vi "Process Incoming Frames.vi"(7 "Incoming Session":refnum<k21>, 8 "error in":errorcluster, 9 "Incoming Signal Info":T4 {"Signal Settings Out"."Protection Configuration"."CRC Channels"."Data Type" items=["Signed", "Unsigned", "IEEE Float"]}, 10 "Incoming RT Data Refs":T2, 11 "Incoming Frame Info In":T1) -> (0 "error out":errorcluster, 1 "Incoming Signal Info Out":T4 {"Signal Settings Out"."Protection Configuration"."CRC Channels"."Data Type" items=["Signed", "Unsigned", "IEEE Float"]}, 3 "Incoming Frame Info Out":T1, 5 "session out":refnum<k21>)   [LabVIEW 2019]
doc: "This example demonstrates receiving automatically converted values of signals, along with the associated timestamp value, using an NI-XNET Signal Input XY session. \n\nThis example can run against the CAN Signal Output XY example, assuming you have a properly terminated CAN cable connected to two CAN ports.\n\nIf you have no database aliases on your system, the example automatically loads the nixnet_example database."
uses:
  Types/Incoming Frame Info.ctl
  SubModules/Frame-Protection-Support/Source/Shared/Types/RT_Incoming_Signal_Info.ctl
  SubModules/Frame-Protection-Support/Source/Shared/Types/RT Exported Signal Settings.ctl
  SubModules/Frame-Protection-Support/Source/Shared/Types/Exported Counter Settings.ctl
  SubModules/Frame-Protection-Support/Source/Engine/Types/RT Protection Configuration.ctl
  SubModules/Frame-Protection-Support/Source/Shared/Types/Protection Type.ctl
  SubModules/Frame-Protection-Support/Source/Shared/Types/XNET Signal Configuration.ctl
  Types/Incoming Signal RT Data References.ctl
  <vilib>/NI/NIVS Inline Async API/_Data Access Engine/Data Access Engine/Types/Write.DVR.ctl
  <vilib>/NI/NIVS Inline Async API/_Data Access Engine/Access Type Classes/Write/Write.lvclass
  <vilib>/NI/NIVS Inline Async API/_Data Access Engine/Access Type Classes/Write/Write.lvclass/Write.ctl
  <vilib>/NI/NIVS Inline Async API/_Data Access Engine/Data Access Engine/Methods/Write.Data.vi
  SubModules/Frame-Protection-Support/Source/Engine/SubVIs/Get Protection Signals.vi
  <vilib>/NI/NIVS Inline Async API/_Data Access Engine/Access Type Classes/Write/Write.ProcessData.vi
  <vilib>/NI/NIVS Inline Async API/_Data Access Engine/Access Type Classes/Write/Write.Buffer.vi
  <vilib>/NI/NIVS Inline Async API/_Data Access Engine/Access Type Classes/Write/Write.Commit.vi
  <vilib>/xnet/xnet.llb/XNET Read (Signal XY).vi
  <vilib>/xnet/xnet.llb/XNET Convert.vi
  <vilib>/xnet/xnet.llb/XNET Convert (Signal to Frame Raw).vi
  <vilib>/NI/NIVS Inline Async API/_Data Access Engine/Data Access Engine/Data Access Engine.lvclass
  <vilib>/NI VeriStand/Custom Device Tools/Custom Device Utility Library/Custom Device Utility Library.lvlib
  SubModules/Frame-Protection-Support/Source/Engine/Protection and Counter Support Engine.lvlib
  SubModules/Frame-Protection-Support/Source/Shared/Protection and Counter Support Shared.lvlib
panel:
  out "data 2":T10(array[cluster])
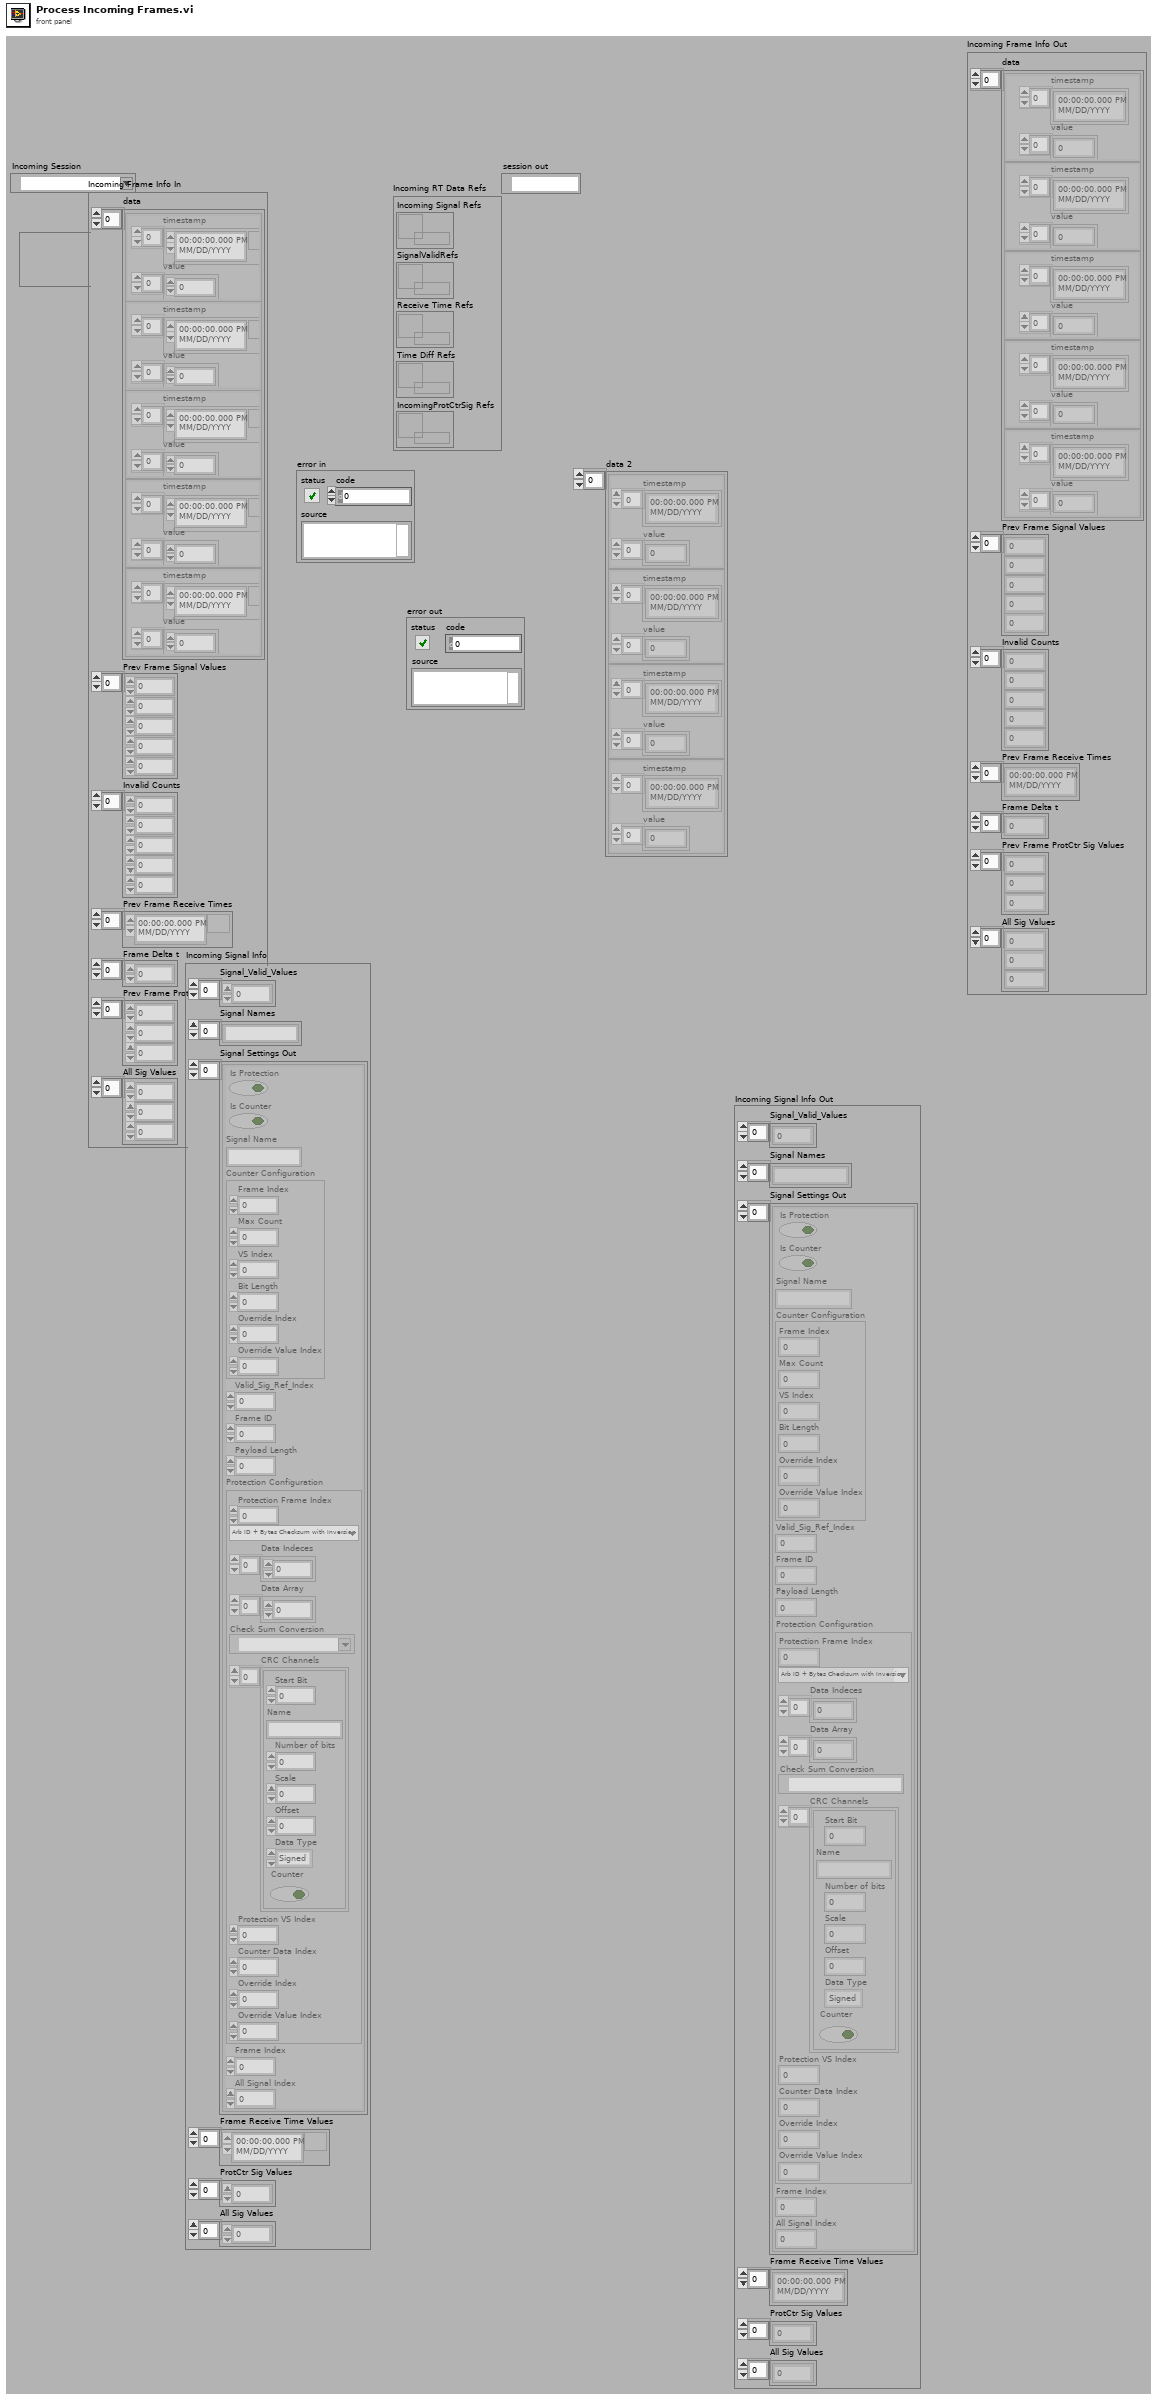
[diagram p1: front panel]
types:
  T1 = typedef "Incoming Frame Info.ctl" = cluster{"data":cluster{"timestamp":timestamp[], "value":dbl[]}[], "Prev Frame Signal Values":dbl[], "Invalid Counts":dbl[], "Prev Frame Receive Times":timestamp[], "Frame Delta t":dbl[], "Prev Frame ProtCtr Sig Values":dbl[], "All Sig Values":dbl[]}
  T2 = typedef "Incoming Signal RT Data References.ctl" = cluster{"Incoming Signal Refs":T3, "SignalValidRefs":T3, "Receive Time Refs":T3, "Time Diff Refs":T3, "IncomingProtCtrSig Refs":T3}
  T3 = typedef "Data Access Engine.lvlib/Data Access Engine.lvclass/Write.DVR.ctl" = refnum<data-value>
  T4 = typedef "RT_Incoming_Signal_Info.ctl" = cluster{"Signal_Valid_Values":dbl[], "Signal Names":string[], "Signal Settings Out":T5[], "Frame Receive Time Values":timestamp[], "ProtCtr Sig Values":dbl[], "All Sig Values":dbl[]}
  T5 = typedef "RT Exported Signal Settings.ctl" = cluster{"Is Protection":bool, "Is Counter":bool, "Signal Name":string, "Counter Configuration":T6, "Valid_Sig_Ref_Index":i32, "Frame ID":u32, "Payload Length":u32, "Protection Configuration":T7, "Frame Index":i32, "All Signal Index":i32}
  T6 = typedef "Protection and Counter Support Shared.lvlib/Exported Counter Settings.ctl" = cluster{"Frame Index":i32, "Max Count":dbl, "VS Index":i32, "Bit Length":i64, "Override Index":i32, "Override Value Index":i32}
  T7 = typedef "Protection and Counter Support Engine.lvlib/RT Protection Configuration.ctl" = cluster{"Protection Frame Index":i32, "Protection Type":T8, "Data Indeces":i32[], "Data Array":dbl[], "Check Sum Conversion":refnum<k21>, "CRC Channels":T9[], "Protection VS Index":i32, "Counter Data Index":i32, "Override Index":i32, "Override Value Index":i32}
  T8 = typedef "Protection and Counter Support Shared.lvlib/Protection Type.ctl" = enum16{"Arb ID + Bytes Checksum with Inversion", "Arb ID + Bytes CRC with Inversion", "Reversed Raw Signal Checksum with Inversion", "Concatenated Two's Compliment"}
  T9 = typedef "Protection and Counter Support Shared.lvlib/XNET Signal Configuration.ctl" = cluster{"Start Bit":i32, "Name":string, "Number of bits":i32, "Scale":dbl, "Offset":dbl, "Data Type":u32, "Counter":bool}
  T10 = cluster{"timestamp":timestamp[], "value":dbl[]}[]
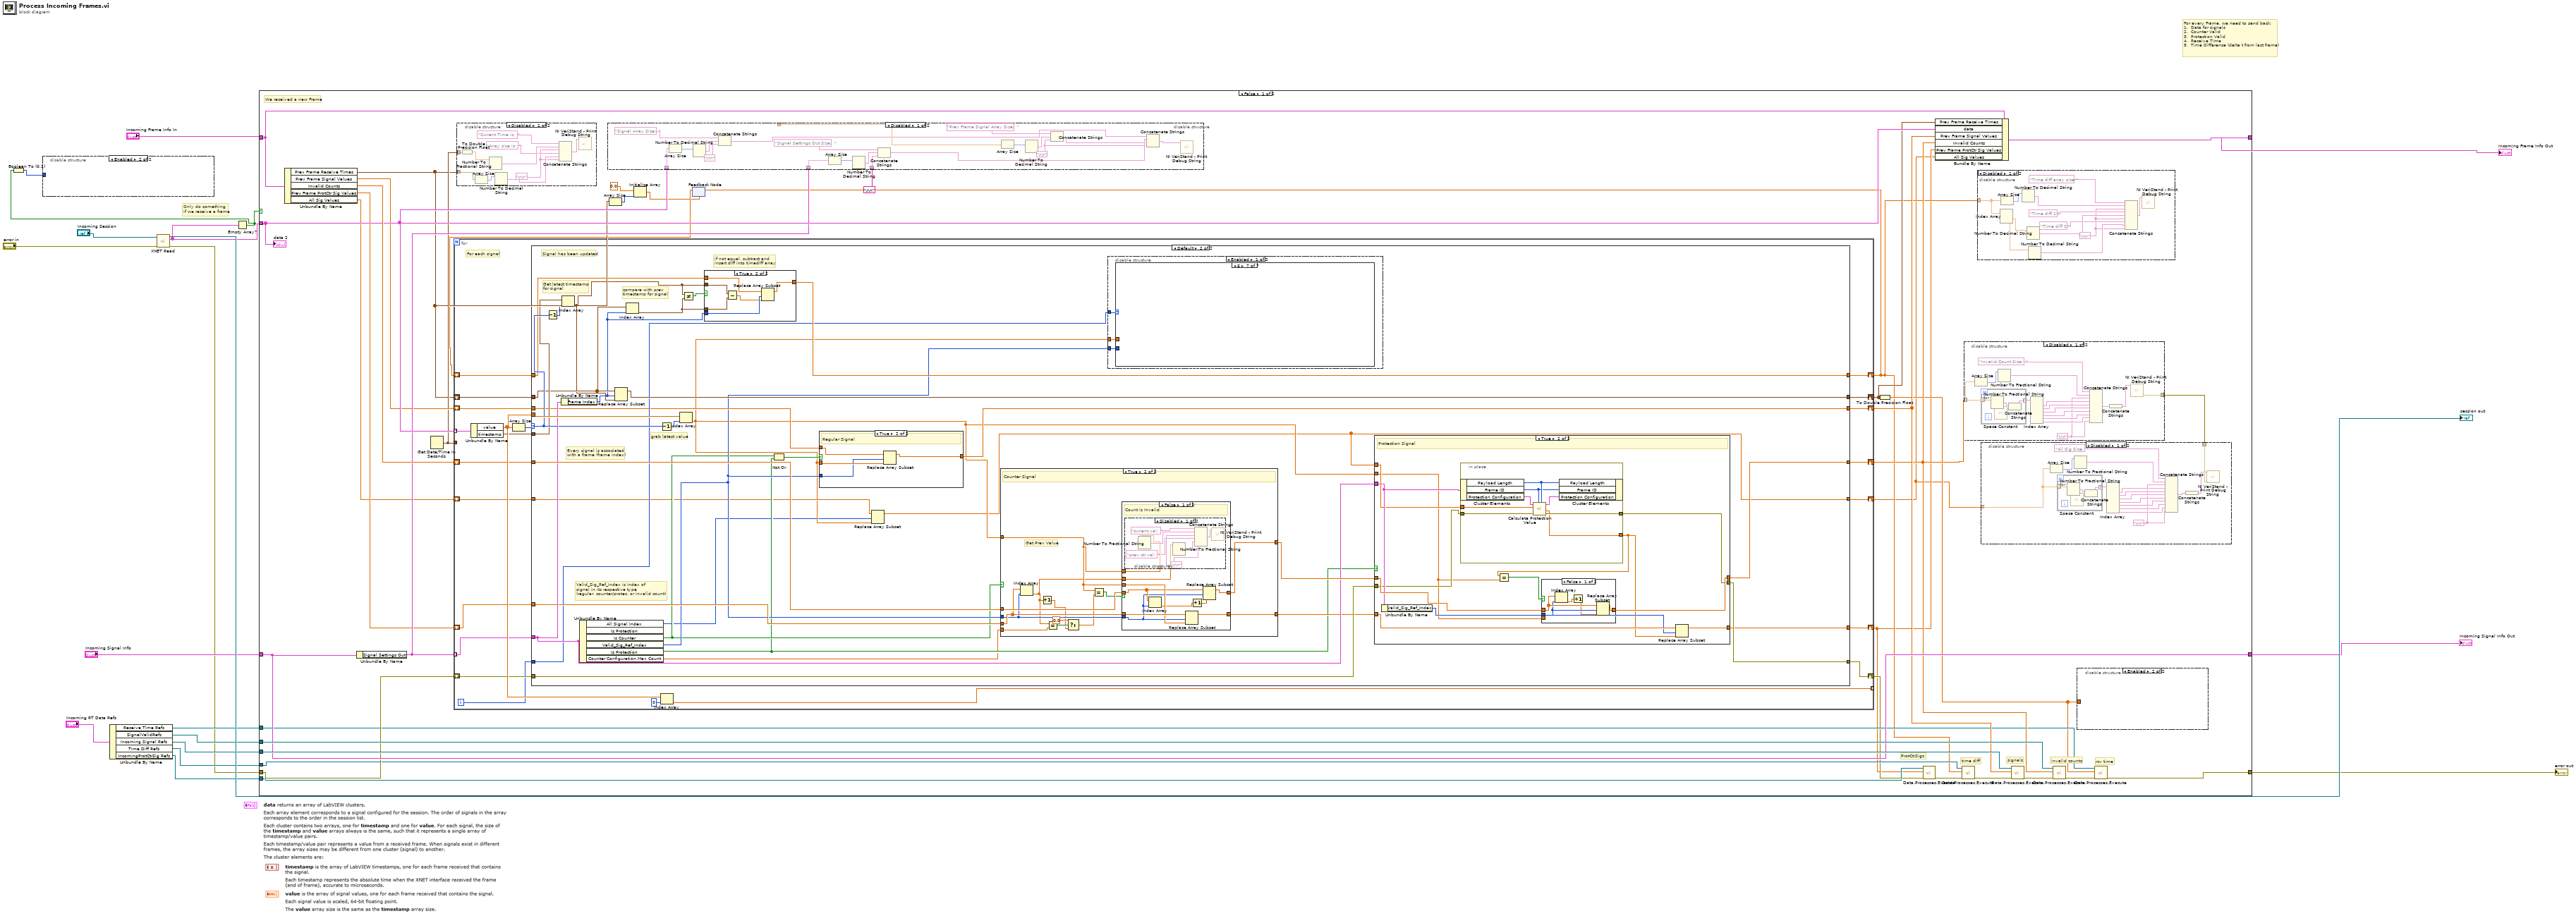
[diagram p0: block diagram]
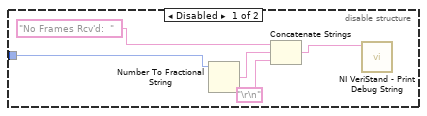
[diagram p2: hidden frame]
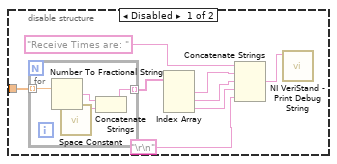
[diagram p7: hidden frame]
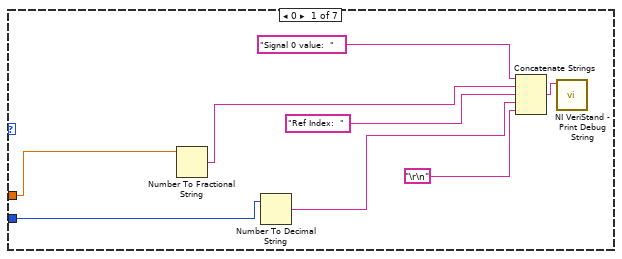
[diagram p11: hidden frame]
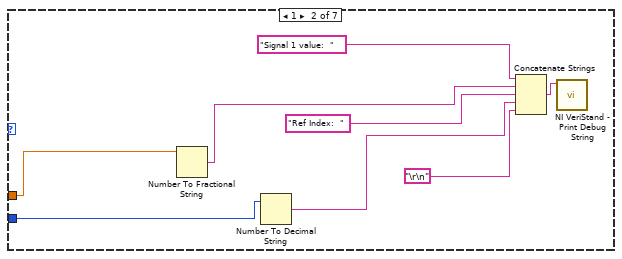
[diagram p12: hidden frame]
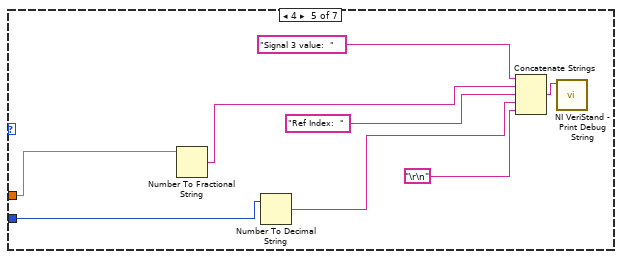
[diagram p15: hidden frame]
diagram:
  # "Only do something\nif we receive a frame"
  # "For every Frame, we need to send back:\n1.  Data for signals\n2.  Counter Valid\n3.  Protection Valid\n4.  Receive Time\n5.  Time Difference (delta t from last frame)"
  n1 = Unbundle By Name("Incoming RT Data Refs") -> ("Receive Time Refs"=w10:T3, "SignalValidRefs"=w9:T3, "Incoming Signal Refs"=w8:T3, "Time Diff Refs"=w4:T3, "IncomingProtCtrSig Refs"=w3:T3)
  n2 = call-poly <vilib>:"XNET Read.vi"("session in"="Incoming Session", "error in (no error)"="error in") -> ("session out"=→"session out":refnum<k21>, "data"=w12:T10, "error out"=w1:errorcluster)  [unwired: 11 out]
  n3 = Empty Array?(array=w12) -> (empty?=w5:bool)
  n4 = Boolean To (0,1)(Boolean=w5) -> (0, 1=w6:i16)
  n5 = disable-structure shown="Enabled" {
    disable-tunnel: w6 -> [w19 _]
    frame Disabled {
      n6 = Number To Fractional String(number=w19) -> (F-format string=w22:string)  [unwired: 3 in]
      n7 = Concatenate Strings("No Frames Rcv'd:  ", w22, "\r\n") -> (w20:string)
      n8 = call <vilib>:"NI VeriStand - Print Debug String.vi"("Message"=w20) -> ()  [unwired: 10 in, 1 out]
    }
    frame Enabled {
    }
  }
  n9 = case shown="False" w5 {
    tunnel: w12 -> [w49 _]
    tunnel: w1 -> [w52 w323]
    tunnel: [w44 w323] -> w15
    tunnel: "Incoming Frame Info In" -> [w55 w322]
    tunnel: [w59 w322] -> w7
    tunnel: w8 -> [w57 _]
    tunnel: w9 -> [w56 _]
    tunnel: "Incoming Signal Info" -> [w54 w321]
    tunnel: [w54 w321] -> w13
    tunnel: w10 -> [w43 _]
    tunnel: w4 -> [w38 _]
    tunnel: w3 -> [w29 _]
    frame False {
      # "ProtCtrSigs"
      # "time diff"
      # "signals"
      # "invalid counts"
      # "rcv time"
      # "We received a new Frame"
      n10 = Unbundle By Name(w55) -> ("Prev Frame Receive Times"=w35:timestamp[], "Prev Frame Signal Values"=w46:dbl[], "Invalid Counts"=w53:dbl[], "Prev Frame ProtCtr Sig Values"=w28:dbl[], "All Sig Values"=w26:dbl[])
      n11 = Unbundle By Name(w54) -> ("Signal Settings Out"=w48:T5[])
      n12 = Get Date/Time In Seconds() -> (seconds since 1Jan1904=w40:timestamp)
      n13 = disable-structure shown="Disabled" {
        disable-tunnel: w40 -> [w116 _]
        disable-tunnel: w35 -> [w115 _]
        frame Disabled {
          w111 = "\r\n"
          n14 = To Double Precision Float(number=w116) -> (double precision float=w117:dbl)
          n15 = Array Size(array=w115) -> (size(s)=w113:i32)
          n16 = Number To Fractional String(number=w117) -> (F-format string=w118:string)  [unwired: 3 in]
          n17 = Number To Decimal String(number=w113) -> (decimal integer string=w112:string)  [unwired: 1 in]
          n18 = Concatenate Strings("Current Time is:  " ("string"), w118, w111, "Array size is:  " ("string"), w112, w111) -> (w119:string)
          n19 = call <vilib>:"NI VeriStand - Print Debug String.vi"("Message"=w119) -> ()  [unwired: 10 in, 1 out]
        }
        frame Enabled {
        }
      }
      n20 = disable-structure shown="Disabled" {
        disable-tunnel: w49 -> [w151 _]
        disable-tunnel: w48 -> [w150 _]
        disable-tunnel: "\r\n" -> [w142 _]
        disable-tunnel: _ -> [w135 _]
        frame Disabled {
          w133 = "\r\n"
          n21 = Array Size(array=w151) -> (size(s)=w147:i32)
          n22 = Number To Decimal String(number=w147) -> (decimal integer string=w148:string)  [unwired: 1 in]
          n23 = Concatenate Strings("Signal Array Size:  ", w148, "\r\n") -> (w140:string)
          n24 = Array Size(array=w150) -> (size(s)=w143:i32)
          n25 = Number To Decimal String(number=w143) -> (decimal integer string=w144:string)  [unwired: 1 in]
          n26 = Concatenate Strings("Signal Settings Out Size:  ", w144, w142) -> (w141:string)
          n27 = Array Size(array=w135) -> (size(s)=w136:i32)
          n28 = Number To Decimal String(number=w136) -> (decimal integer string=w137:string)  [unwired: 1 in]
          n29 = Concatenate Strings("Prev Frame Signal Array Size:  ", w137, w133) -> (w134:string)
          n30 = Concatenate Strings(w140, w141, w134, w133) -> (w139:string)
          n31 = call <vilib>:"NI VeriStand - Print Debug String.vi"("Message"=w139) -> ()  [unwired: 10 in, 1 out]
        }
        frame Enabled {
        }
      }
      n32 = Array Size(array=w35) -> (size(s)=w36:i32)
      n33 = Initialize Array(0.0, w36) -> (w32:dbl[])
      n34 = feedback #1(w32) -> (w33:dbl[])
      n35 = for {
        tunnel: w49 -> [w173] mode=indexing
        shift-right: [w170] -> w51
        shift-left: w46 -> [w171]
        tunnel: [w167] -> _ mode=indexing
        tunnel: w48 -> [w166] mode=indexing
        shift-right: [w164] -> w50
        shift-left: w53 -> [w165]
        shift-right: [w162] -> w31
        shift-left: w52 -> [w163]
        shift-right: [w160] -> w42
        shift-left: w35 -> [w161]
        tunnel: w40 -> [_]
        shift-right: [w159] -> w34
        shift-left: w33 -> [w158]
        shift-right: [w155] -> w27
        shift-left: w28 -> [w156]
        shift-right: [w152] -> w24
        shift-left: w26 -> [w153]
        i -> [w154]
        # "For each signal"
        n36 = Unbundle By Name(w173) -> ("value"=w169:dbl[], "timestamp"=w157:timestamp[])
        n37 = Array Size(array=w169) -> (size(s)=w172:i32)
        n38 = case shown="Default" w172 {
          selector: w172 -> [_ w205]
          tunnel: w157 -> [_ w203]
          tunnel: w171 -> [w180 w191]
          tunnel: [w180 w189] -> w170
          tunnel: w169 -> [_ w214]
          tunnel: w166 -> [_ w207]
          tunnel: w165 -> [w179 w212]
          tunnel: [w179 w208] -> w164
          tunnel: w163 -> [w178 w211]
          tunnel: [w178 w210] -> w162
          tunnel: w161 -> [w177 w202]
          tunnel: [w177 w206] -> w160
          tunnel: [w176 w197] -> w159
          tunnel: w158 -> [w176 w199]
          tunnel: w156 -> [w175 w195]
          tunnel: [w175 w193] -> w155
          tunnel: w154 -> [_ w192]
          tunnel: w153 -> [w174 w184]
          tunnel: [w174 w181] -> w152
          frame 0 {
            # "The signal has not been updated, so\npass through previous value"
          }
          frame Default {
            # "Valid_Sig_Ref_Index is index of \nsignal in its respective type \n(regular, counter/protec, or invalid count)"
            # "if not equal, subtract and\ninsert diff into timediff array"
            # "compare with prev\ntimestamp for signal"
            # "Get latest timestamp\nfor signal"
            # "Signal has been updated"
            # "Every signal is associated \nwith a frame (frame index)"
            # "grab latest value"
            n39 = Decrement(x=w205) -> (x-1=w204:i32)
            n40 = Unbundle By Name(w207) -> ("Frame Index"=w196:i32)
            n41 = Index Array(array=w203, index=w204) -> (element=w198:timestamp)
            n42 = Unbundle By Name(w207) -> ("All Signal Index"=w182:i32, "Is Counter"=w188:bool, "Valid_Sig_Ref_Index"=w190:i32, "Is Protection"=w187:bool, "Counter Configuration.Max Count"=w185:dbl)  [unwired: 1 out]
            n43 = Replace Array Subset(array=w202, new element=w198, index=w196) -> (w206:timestamp[])
            n44 = Index Array(array=w202, index=w196) -> (element=w200:timestamp)
            n45 = Decrement(x=w205) -> (x-1=w213:i32)
            n46 = Index Array(array=w214, index=w213) -> (element=w183:dbl)
            n47 = Not Equal?(x=w198, y=w200) -> (x != y?=w201:bool)
            n48 = case shown="True" w201 {
              tunnel: w198 -> [_ w253]
              tunnel: w200 -> [_ w252]
              tunnel: w196 -> [_ w251]
              tunnel: w199 -> [w247 w249]
              tunnel: [w247 w248] -> w197
              frame False {
              }
              frame True {
                n49 = Subtract(x=w253, y=w252) -> (x-y=w250:dbl)
                n50 = Replace Array Subset(array=w249, new element=w250, index=w251) -> (w248:dbl[])
              }
            }
            n51 = Not Or(1:w187, 2:w188) -> (0:w186:bool)
            n52 = case shown="True" w186 {
              tunnel: w191 -> [w215 w219]
              tunnel: w183 -> [_ w218]
              tunnel: w190 -> [_ w217]
              tunnel: [w215 w216] -> w189
              frame False {
              }
              frame True {
                # "Regular Signal"
                n53 = Replace Array Subset(array=w219, new element=w218, index=w217) -> (w216:dbl[])
              }
            }
            n54 = Replace Array Subset(array=w184, new element=w183, index=w182) -> (w181:dbl[])
            n55 = case shown="True" w188 {
              tunnel: w183 -> [_ w286]
              tunnel: w212 -> [w284 w297]
              tunnel: w190 -> [_ w293]
              tunnel: [w284 w296] -> w209
              tunnel: w195 -> [w283 w294]
              tunnel: [w283 w295] -> w194
              tunnel: w185 -> [_ w292]
              frame False {
              }
              frame True {
                # "Get Prev Value"
                # "Counter Signal"
                n56 = Index Array(array=w294, index=w293) -> (element=w285:dbl)
                n57 = Increment(x=w285) -> (x+1=w289:dbl)
                n58 = Equal?(x=w285, y=w292) -> (x = y?=w291:bool)
                n59 = Select(t=0.0, s=w291, f=w289) -> (s? t:f=w288:dbl)
                n60 = Equal?(x=w286, y=w288) -> (x = y?=w287:bool)
                n61 = case shown="False" w287 {
                  tunnel: w297 -> [w304 w320]
                  tunnel: [w300 w320] -> w296
                  tunnel: w286 -> [w306 w319]
                  tunnel: [w305 w318] -> w295
                  tunnel: w294 -> [w307 w317]
                  tunnel: w293 -> [w303 w316]
                  tunnel: w286 -> [w299 _]
                  tunnel: w285 -> [w298 _]
                  frame False {
                    # "Count is Invalid"
                    n62 = disable-structure shown="Disabled" {
                      disable-tunnel: w299 -> [w312 _]
                      disable-tunnel: w298 -> [w311 _]
                      frame Disabled {
                        w308 = "\r\n"
                        n63 = Number To Fractional String(number=w312) -> (F-format string=w313:string)  [unwired: 3 in]
                        n64 = Number To Fractional String(number=w311) -> (F-format string=w309:string)  [unwired: 3 in]
                        n65 = Concatenate Strings("current val:  ", w313, w308, "prev ctr val:  ", w309, w308) -> (w315:string)
                        n66 = call <vilib>:"NI VeriStand - Print Debug String.vi"("Message"=w315) -> ()  [unwired: 10 in, 1 out]
                      }
                      frame Enabled {
                      }
                    }
                    n67 = Index Array(array=w304, index=w303) -> (element=w302:dbl)
                    n68 = Replace Array Subset(array=w307, new element=w306, index=w303) -> (w305:dbl[])
                    n69 = Increment(x=w302) -> (x+1=w301:dbl)
                    n70 = Replace Array Subset(array=w304, new element=w301, index=w303) -> (w300:dbl[])
                  }
                  frame True {
                    # "Count is Valid"
                    n71 = Replace Array Subset(array=w317, new element=w319, index=w316) -> (w318:dbl[])
                  }
                }
              }
            }
            n72 = disable-structure shown="Enabled" {
              disable-tunnel: w192 -> [w222 _]
              disable-tunnel: w183 -> [w221 _]
              disable-tunnel: w190 -> [w220 _]
              frame Enabled {
                n73 = case shown="6" w222 {
                  tunnel: w221 -> [w227 w235 _ _ w243 _ _]
                  tunnel: w220 -> [w224 w232 _ _ w240 _ _]
                  frame 0 {
                    n74 = Number To Fractional String(number=w227) -> (F-format string=w226:string)  [unwired: 3 in]
                    n75 = Number To Decimal String(number=w224) -> (decimal integer string=w223:string)  [unwired: 1 in]
                    n76 = Concatenate Strings("Signal 0 value:  " ("string"), w226, "Ref Index:  " ("string"), w223, "\r\n") -> (w230:string)
                    n77 = call <vilib>:"NI VeriStand - Print Debug String.vi"("Message"=w230) -> ()  [unwired: 10 in, 1 out]
                  }
                  frame 1 {
                    n78 = Number To Fractional String(number=w235) -> (F-format string=w234:string)  [unwired: 3 in]
                    n79 = Number To Decimal String(number=w232) -> (decimal integer string=w231:string)  [unwired: 1 in]
                    n80 = Concatenate Strings("Signal 1 value:  " ("string"), w234, "Ref Index:  " ("string"), w231, "\r\n") -> (w238:string)
                    n81 = call <vilib>:"NI VeriStand - Print Debug String.vi"("Message"=w238) -> ()  [unwired: 10 in, 1 out]
                  }
                  frame 2 {
                  }
                  frame 3, Default {
                  }
                  frame 4 {
                    n82 = Number To Fractional String(number=w243) -> (F-format string=w242:string)  [unwired: 3 in]
                    n83 = Number To Decimal String(number=w240) -> (decimal integer string=w239:string)  [unwired: 1 in]
                    n84 = Concatenate Strings("Signal 3 value:  " ("string"), w242, "Ref Index:  " ("string"), w239, "\r\n") -> (w246:string)
                    n85 = call <vilib>:"NI VeriStand - Print Debug String.vi"("Message"=w246) -> ()  [unwired: 10 in, 1 out]
                  }
                  frame 5 {
                  }
                  frame 6 {
                  }
                }
              }
              frame Disabled {
              }
            }
            n86 = case shown="True" w187 {
              tunnel: w211 -> [w256 w261]
              tunnel: [w256 w262] -> w210
              tunnel: w207 -> [_ w263]
              tunnel: w209 -> [w255 w268]
              tunnel: [w255 w267] -> w208
              tunnel: w183 -> [_ w258]
              tunnel: w194 -> [w254 w266]
              tunnel: [w254 w264] -> w193
              tunnel: w181 -> [_ w260]
              frame False {
              }
              frame True {
                # "Protection Signal"
                n87 = Unbundle By Name(w263) -> ("Valid_Sig_Ref_Index"=w265:i32)
                n88 = in-place {
                  in-place-border: w261 -> [w282]
                  in-place-border: [w278] -> w262
                  in-place-border: w260 -> [w276]
                  in-place-border: [w275] -> w259
                  n89 = in-place-cluster #2(w263) -> ("Payload Length"=w281:u32, "Frame ID"=w280:u32, "Protection Configuration"=w279:T7)
                  n90 = call "Calculate Protection Value.vi"("Payload Length"=w281, "Frame ID"=w280, "error in (no error)"=w282, "Frame.Data in"=w276, "Protection Configuration in"=w279) -> ("error out"=w278:errorcluster, "Protection Value"=w275:dbl, "Protection Configuration out"=w277:T7)  [unwired: 3 in, 1 out]
                  n91 = in-place-cluster #2("Payload Length"=w281, "Frame ID"=w280, "Protection Configuration"=w277) -> ()  [unwired: 1 out]
                }
                n92 = Equal?(x=w259, y=w258) -> (x = y?=w257:bool)
                n93 = case shown="False" w257 {
                  tunnel: w268 -> [w272 w274]
                  tunnel: [w273 w274] -> w267
                  tunnel: w265 -> [w271 _]
                  tunnel: w258 -> [_ _]
                  frame False {
                    n94 = Index Array(array=w272, index=w271) -> (element=w270:dbl)
                    n95 = Increment(x=w270) -> (x+1=w269:dbl)
                    n96 = Replace Array Subset(array=w272, new element=w269, index=w271) -> (w273:dbl[])
                  }
                  frame True {
                  }
                }
                n97 = Replace Array Subset(array=w266, new element=w259, index=w265) -> (w264:dbl[])
              }
            }
          }
        }
        n98 = Index Array(array=w169, index=0) -> (element=w167:dbl)
      }
      n99 = feedback-in #1(w34) -> ()
      n100 = To Double Precision Float(number=w42) -> (double precision float=w41:dbl[])
      n101 = call-poly <vilib>:"Data.Processes.Execute.vi"("error in (no error)"=w31, "Values"=w27, "Ref"=w29) -> ("error out"=w30:errorcluster)  [unwired: 8 in]
      n102 = Bundle By Name(cluster=w55, "Prev Frame Receive Times"=w42, "data"=w49, "Prev Frame Signal Values"=w51, "Invalid Counts"=w50, "Prev Frame ProtCtr Sig Values"=w27, "All Sig Values"=w24) -> (w59:T1)
      n103 = call-poly <vilib>:"Data.Processes.Execute.vi"("error in (no error)"=w30, "Values"=w34, "Ref"=w38) -> ("error out"=w39:errorcluster)  [unwired: 8 in]
      n104 = disable-structure shown="Disabled" {
        disable-tunnel: w50 -> [w94 _]
        disable-tunnel: [w80 _] -> w25
        frame Disabled {
          w83 = "\r\n"
          n105 = Array Size(array=w94) -> (size(s)=w93:i32)
          n106 = for {
            tunnel: w94 -> [w96] mode=indexing
            tunnel: [w95] -> w90 mode=indexing
            n107 = Number To Fractional String(number=w96) -> (F-format string=w98:string)  [unwired: 3 in]
            n108 = call <vilib>:"Space Constant.vi"() -> ("String"=w97:string)
            n109 = Concatenate Strings(w98, w97) -> (w95:string)
          }
          n110 = Number To Fractional String(number=w93) -> (F-format string=w91:string)  [unwired: 3 in]
          n111 = Index Array(array=w90) -> (element #1=w89:string, element #2=w88:string, element #3=w87:string, element #4=w86:string, element #5=w85:string, element #6=w84:string)  [unwired: 6 in]
          n112 = Concatenate Strings("Invalid Count Size:  ", w91, w83, w89, w88, w87, w86, w85, w84, w83) -> (w82:string)
          n113 = Concatenate Strings(w82) -> (w81:string)
          n114 = call <vilib>:"NI VeriStand - Print Debug String.vi"("Message"=w81) -> ("error out"=w80:errorcluster)  [unwired: 10 in]
        }
        frame Enabled {
        }
      }
      n115 = disable-structure shown="Disabled" {
        disable-tunnel: w34 -> [w106 _]
        frame Disabled {
          w99 = "\r\n"
          n116 = Index Array(array=w106) -> (element #1=w105:dbl, element #2=w104:dbl)  [unwired: 2 in]
          n117 = Array Size(array=w106) -> (size(s)=w108:i32)
          n118 = Number To Decimal String(number=w108) -> (decimal integer string=w107:string)  [unwired: 1 in]
          n119 = Number To Decimal String(number=w105) -> (decimal integer string=w102:string)  [unwired: 1 in]
          n120 = Number To Decimal String(number=w104) -> (decimal integer string=w100:string)  [unwired: 1 in]
          n121 = Concatenate Strings("Time diff array size:" ("string"), w107, w99, "Time diff 1:" ("string"), w102, w99, "Time diff 2:" ("string"), w100, w99) -> (w109:string)
          n122 = call <vilib>:"NI VeriStand - Print Debug String.vi"("Message"=w109) -> ()  [unwired: 10 in, 1 out]
        }
        frame Enabled {
        }
      }
      n123 = disable-structure shown="Disabled" {
        disable-tunnel: w25 -> [w62 _]
        disable-tunnel: w24 -> [w61 _]
        frame Disabled {
          w65 = "\r\n"
          n124 = Array Size(array=w61) -> (size(s)=w75:i32)
          n125 = for {
            tunnel: w61 -> [w77] mode=indexing
            tunnel: [w76] -> w72 mode=indexing
            n126 = Number To Fractional String(number=w77) -> (F-format string=w79:string)  [unwired: 3 in]
            n127 = call <vilib>:"Space Constant.vi"() -> ("String"=w78:string)
            n128 = Concatenate Strings(w79, w78) -> (w76:string)
          }
          n129 = Number To Fractional String(number=w75) -> (F-format string=w73:string)  [unwired: 3 in]
          n130 = Index Array(array=w72) -> (element #1=w71:string, element #2=w70:string, element #3=w69:string, element #4=w68:string, element #5=w67:string, element #6=w66:string, element #7=w60:string)  [unwired: 7 in]
          n131 = Concatenate Strings("All Sig Size:  ", w73, w65, w71, w70, w69, w68, w67, w66, w60, w65) -> (w64:string)
          n132 = Concatenate Strings(w64) -> (w63:string)
          n133 = call <vilib>:"NI VeriStand - Print Debug String.vi"("error in (no error)"=w62, "Message"=w63) -> ()  [unwired: 9 in, 1 out]
        }
        frame Enabled {
        }
      }
      n134 = call-poly <vilib>:"Data.Processes.Execute.vi"("error in (no error)"=w39, "Values"=w51, "Ref"=w57) -> ("error out"=w58:errorcluster)  [unwired: 8 in]
      n135 = call-poly <vilib>:"Data.Processes.Execute.vi"("error in (no error)"=w58, "Values"=w50, "Ref"=w56) -> ("error out"=w45:errorcluster)  [unwired: 8 in]
      n136 = disable-structure shown="Enabled" {
        disable-tunnel: w41 -> [w127 _]
        frame Disabled {
          n137 = for {
            tunnel: w127 -> [w130] mode=indexing
            tunnel: [w129] -> w126 mode=indexing
            n138 = Number To Fractional String(number=w130) -> (F-format string=w132:string)  [unwired: 3 in]
            n139 = call <vilib>:"Space Constant.vi"() -> ("String"=w131:string)
            n140 = Concatenate Strings(w132, w131) -> (w129:string)
          }
          n141 = Index Array(array=w126) -> (element #1=w125:string, element #2=w124:string, element #3=w123:string)  [unwired: 3 in]
          n142 = Concatenate Strings("Receive Times are: " ("string"), w125, w124, w123, "\r\n") -> (w121:string)
          n143 = call <vilib>:"NI VeriStand - Print Debug String.vi"("Message"=w121) -> ()  [unwired: 10 in, 1 out]
        }
        frame Enabled {
        }
      }
      n144 = call-poly <vilib>:"Data.Processes.Execute.vi"("error in (no error)"=w45, "Values"=w41, "Ref"=w43) -> ("error out"=w44:errorcluster)  [unwired: 8 in]
      "data 2" <- w49
    }
    frame True {
      # "No Frame Received"
    }
  }
  "error out" <- w15
  "Incoming Signal Info Out" <- w13
  "Incoming Frame Info Out" <- w7
